vi "HMI Test.vi"() -> ()   [LabVIEW 2023]
uses:
  Types/Setpoints.ctl
  Types/Power Function.ctl
  Types/Range.ctl
panel:
  out "Current Range":T1 caption="RANGE"
  out "Voltage Range":T1 caption="RANGE"
  out "Charging":bool caption="CHARGE"
  out "Discharging":bool caption="DISCHARGE"
  in  "Module Selection":i16(ring)=-1 caption="MODULE" items=["NONE"=-1, "HPS-17000"=0, "Simulated"=1]
  out "EMO Indicator":u16(ring)
  in  "Start Logging":bool
  out "Function":T2=enum."STANDBY" caption="FUNCTION"
  out "MODE":u16(ring)=193 items=["UNKNOWN"=0, "CONSTANT VOLTAGE"=1, "CONSTANT CURRENT"=2, "INTERNAL RECIRCULATION"=193]
  in  "PMOD Clear":bool
  out "Status Message":string
  in  "PMOD Reserve":bool
  in  "PMOD Connect":bool
  out "Fault Message":string
  in  "Acknowledge Faults":bool
  out "Power Maximum":dbl caption="MAX"
  out "Power Minimum":dbl caption="MIN"
  out "Current Maximum":dbl caption="MAX"
  out "Current Minimum":dbl caption="MIN"
  out "Voltage Maximum":dbl caption="MAX"
  out "Voltage Minimum":dbl caption="MIN"
  in  "Main Tab Control":T3(tab)=enum."CONTROL"
  out "XY Graph":T4(graph)
  in  "Use Local Time":bool caption="LOCAL TIME"
  in  "High Speed":bool caption="HIGH SPEED"
  in  "Pause Chart":bool
  in  "Save Chart":bool
  in  "Erase Chart":bool
  out "Module Plugin Directory":path caption="MODULE PLUGIN DIRECTORY"
  in  "Profile Step dT (ns)":i64=10000 caption="PROFILE STEP TIME (ns)"
  in  "Graph Samples":u32=10000 caption="CHART SAMPLES"
  in  "Graph Data Decimation":i32=100 caption="CHART DECIMATION"
  in  "Log File Directory":path caption="LOG FILE DIRECTORY"
  in  "Power Module Plugins":i32(listbox) caption="POWER MODULE PLUGINS"
  in  "Apply Slew Rates":bool
  in  "Slew Rates":T5={"Voltage Inc. [V/sec]"=inf, "Voltage Dec. [V/sec]"=inf, "Current Inc. [A/sec]"=inf, "Current Dec. [A/sec]"=inf, "Resistance Inc. [Ohms/sec]"=inf, "Resistance Dec. [Ohms/sec]"=inf} caption="SLEW RATES"
  in  "Output":bool caption="OUTPUT"
  in  "Apply Limits":bool
  in  "Limits":T6 caption="LIMITS"
  in  "Apply Setpoints":bool
  in  "Setpoints":T7 caption="SETPOINTS"
  in  "Energize":bool caption="ENERGIZE"
  in  "Apply Mode & Range":bool
  in  "Mode & Range":cluster{"Mode":u16, "Range":u16}={"Mode"=193, "Range"=1} caption="MODE | RANGE" {"Range" items=["Low Voltage"=1, "High Voltage"=2]; "Mode" items=["Constant Voltage"=1, "Constant Current"=2, "Internal Recirculation"=193, "V_VCC"=33, "V_VCC_R"=34, "V_VCC_RADJ"=35]}
  out "Mini Chart":dbl[][](graph)
  in  "CSV Profile 2":path caption="CSV PROFILE"
  in  "Start Profile":bool
  out "CSV Profile":waveform(dbl)[](graph)
  in  "Battery Cells in Parallel":u16=1 caption="# Cells in Parallel"
  in  "Battery Cells in Series":u16=100 caption="# Cells in Series"
  in  "Reset Battery Simulation":bool
  in  "Battery Model Parameters":T8={"Parameter Set"="Chen2020", "Model Type"="SPMe"}
  in  "Use Battery Model":bool caption="ENABLE BATTERY SIMULATION"
  in  "Battery Simulation Parameters":T9={"EIS Start Frequency"=1, "EIS Stop Frequency"=0.0015, "EIS Stop Frequency 2"=0.001, "EIS Stop Frequency 3"=2500.0, "EIS Stop Frequency 4"=0.0008, "EIS Stop Frequency 5"=40000.0, "EIS Stop Frequency 6"=5.0, "EIS Stop Frequency 7"=4.2, "EIS Stop Frequency 8"=3.0} {"EIS Start Frequency" min=1 max=2}
  in  "Launch Battery Simulation":bool
  in  "Toggle EIS Profile":bool
  in  "Generate EIS Profile":bool
  in  "EIS Save & Load Profile":bool
  in  "Generate EIS Report":bool
  in  "EIS Parameters":T10={"EIS Mode"=2, "EIS DC Potential"=650.0, "EIS Start Frequency"=1000.0, "EIS Stop Frequency"=500.0, "EIS Delta Frequency"=100.0, "EIS DC Current"=0.0, "AC Signal (mV/mA RMS)"=20.0, "Cycles at Frequency"=5.0, "EIS AC Step Delay"=1.0} {"EIS Mode" items=["Voltage (PEIS)"=1, "Current (GEIS)"=2]}
  in  "Toggle HPPC Profile":bool
  in  "Generate HPPC Profile":bool
  in  "HPPC Save & Load Profile":bool
  in  "Generate HPPC Report":bool
  in  "HPPC Parameters":T11={"Initial SoC (%)"=75.0, "Pulse Mode"=2, "Pulse Current (A)"=10.0, "Pulse Duration (S)"=10.0} {"Pulse Mode" items=["Discharge"=1, "Charge"=2]; "Initial SoC (%)" min=0.0 max=100.0}
  in  "TDMS Viewer":bool
  out "Fault":bool caption="FAULT"
  out "Output Enabled":bool caption="OUTPUT ENABLED"
  out "Output Disabled":bool caption="OUTPUT DISABLED"
  out "System Power":bool caption="SYSTEM ENERGIZED"
  out "POWER":dbl(knob) caption="Gauge" scale=150.0..-150.0
  out "CURRENT":dbl(knob) caption="Gauge" scale=480.0..-480.0
  out "VOLTAGE":dbl(knob) caption="Gauge"
  # "-"
  # "-"
  # "OFF               ON"
  # "OFF               ON"
  # "#TODO\n\nPYTHON ENVIRONMENT DETAILS\n\nLABVIEW RUN TIME ENVIRONMENT DETAILS\n\nVOLTA CONTROL SUITE DETAILS\n\nVOLTA CONTROL SUITE CHM OR HELP MANUAL"
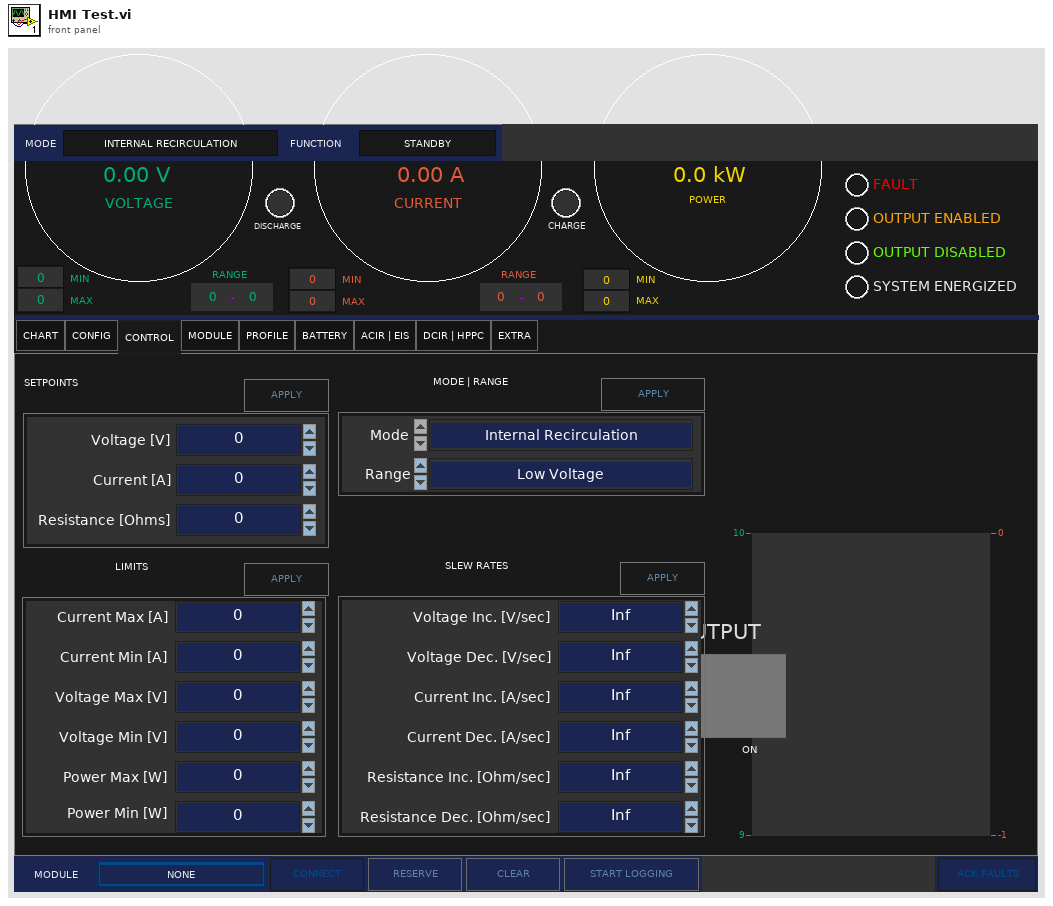
[diagram p1: front panel]
types:
  T1 = typedef "Range.ctl" = cluster{"min":dbl, "max":dbl}
  T2 = typedef "Power Function.ctl" = enum16{"REGEN (LOAD)", "STANDBY", "SUPPLY (SOURCE)"}
  T3 = enum32{"CHART", "CONFIG", "CONTROL", "MODULE", "PROFILE", "BATTERY", "ACIR | EIS", "DCIR | HPPC", "EXTRA"}
  T4 = cluster{"timestamp":dbl[], "setpoint current":dbl[]}[]
  T5 = cluster{"Voltage Inc. [V/sec]":sgl, "Voltage Dec. [V/sec]":sgl, "Current Inc. [A/sec]":sgl, "Current Dec. [A/sec]":sgl, "Resistance Inc. [Ohms/sec]":sgl, "Resistance Dec. [Ohms/sec]":sgl}
  T6 = cluster{"Current Max Limit":sgl, "Current Min Limit":sgl, "Voltage Max Limit":sgl, "Voltage Min Limit":sgl, "Power Max Limit":sgl, "Power Min Limit":sgl}
  T7 = typedef "Setpoints.ctl" = cluster{"Voltage":dbl, "Current":dbl, "Resistance [Ohms]":dbl}
  T8 = cluster{"Parameter Set":string, "Model Type":string}
  T9 = cluster{"EIS Start Frequency":u8, "EIS Stop Frequency":dbl, "EIS Stop Frequency 2":dbl, "EIS Stop Frequency 3":dbl, "EIS Stop Frequency 4":dbl, "EIS Stop Frequency 5":dbl, "EIS Stop Frequency 6":dbl, "EIS Stop Frequency 7":dbl, "EIS Stop Frequency 8":dbl}
  T10 = cluster{"EIS Mode":u16, "EIS DC Potential":dbl, "EIS Start Frequency":dbl, "EIS Stop Frequency":dbl, "EIS Delta Frequency":dbl, "EIS DC Current":dbl, "AC Signal (mV/mA RMS)":dbl, "Cycles at Frequency":dbl, "EIS AC Step Delay":dbl}
  T11 = cluster{"Initial SoC (%)":dbl, "Pulse Mode":u16, "Pulse Current (A)":dbl, "Pulse Duration (S)":dbl}
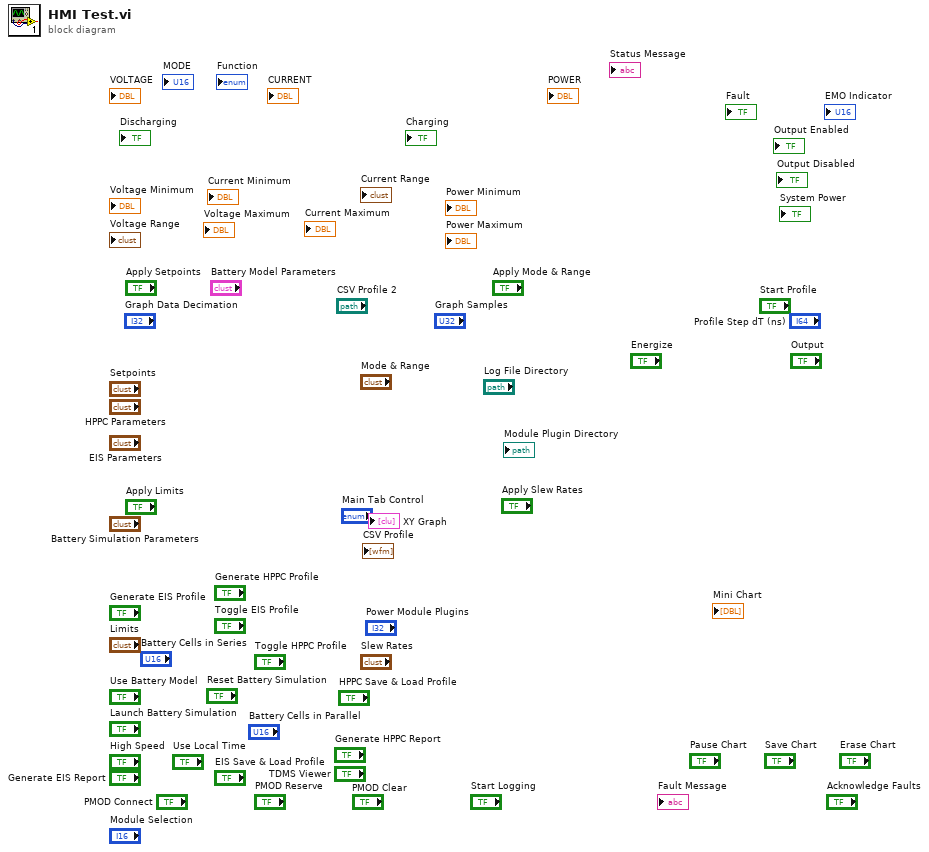
[diagram p0: block diagram]
diagram:
